vi "SeCrTs-ACC_Read_P3.vi"(7 "Data FIFO Ref":T1, 8 "error in (no error)":errorcluster, 9 "number of samples per channel":i32, 10 "ACC_Task":refnum<k21>) -> (0 "error out":errorcluster, 2 "task out":refnum<k21>)   [LabVIEW 2022 SP3]
uses:
  RT Controls/SeCrTs-Data FIFO.ctl
  <vilib>/Platform/TimedLoop/XDataNode/timing_clust.ctl
  <vilib>/Platform/TimedLoop/XDataNode/nitl_modes.ctl
  <vilib>/Platform/TimedLoop/XDataNode/wakeup.ctl
  <vilib>/DAQmx/read.llb/DAQmx Read (Analog 1D Wfm NChan NSamp).vi
  <vilib>/DAQmx/miscellaneous.llb/DAQmx Fill In Error Info.vi
  <vilib>/platform/TimedLoop/XDataNode/XDataNode.xnode
  <vilib>/Platform/TimedLoop/XDataNode/XDNodeRunTimeDep.lvlib
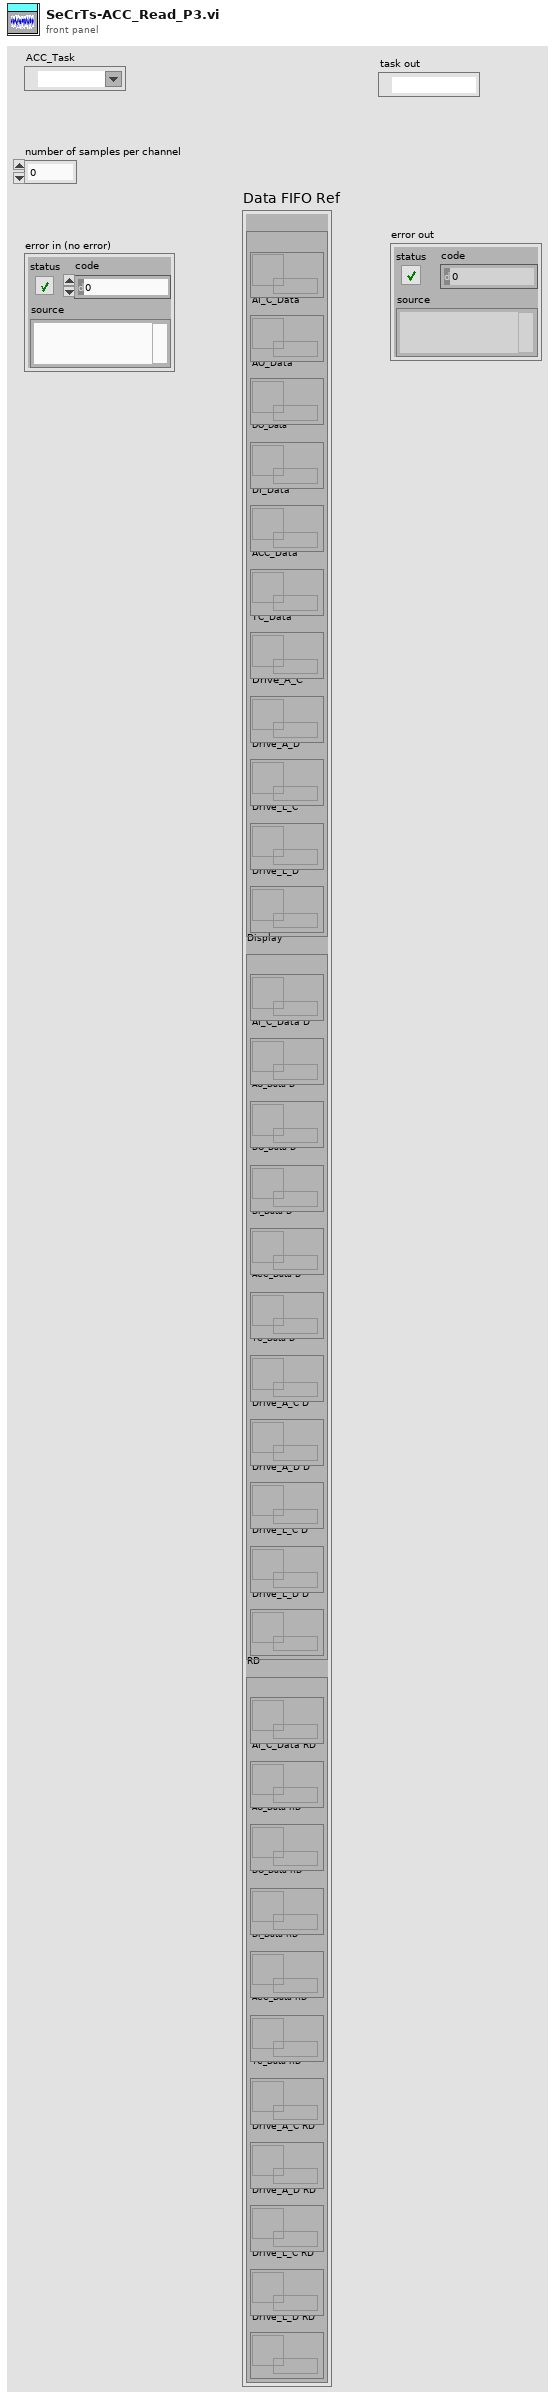
[diagram p1: front panel]
types:
  T1 = typedef "SeCrTs-Data FIFO.ctl" = cluster{"Control":cluster{"AI_V_Data":refnum<queue>, "AI_C_Data":refnum<queue>, "AO_Data":refnum<queue>, "DO_Data":refnum<queue>, "DI_Data":refnum<queue>, "ACC_Data":refnum<queue>, "TC_Data":refnum<queue>, "Drive_A_C":refnum<queue>, "Drive_A_D":refnum<queue>, "Drive_L_C":refnum<queue>, "Drive_L_D":refnum<queue>}, "Display":cluster{"AI_V_Data D":refnum<queue>, "AI_C_Data D":refnum<queue>, "AO_Data D":refnum<queue>, "DO_Data D":refnum<queue>, "DI_Data D":refnum<queue>, "ACC_Data D":refnum<queue>, "TC_Data D":refnum<queue>, "Drive_A_C D":refnum<queue>, "Drive_A_D D":refnum<queue>, "Drive_L_C D":refnum<queue>, "Drive_L_D D":refnum<queue>}, "RD":cluster{"AI_V_Data RD":refnum<queue>, "AI_C_Data RD":refnum<queue>, "AO_Data RD":refnum<queue>, "DO_Data RD":refnum<queue>, "DI_Data RD":refnum<queue>, "ACC_Data RD":refnum<queue>, "TC_Data RD":refnum<queue>, "Drive_A_C RD":refnum<queue>, "Drive_A_D RD":refnum<queue>, "Drive_L_C RD":refnum<queue>, "Drive_L_D RD":refnum<queue>}}
  T2 = typedef "XDNodeRunTimeDep.lvlib/timing_clust.ctl" = cluster{"Expected End [f-1]":u64, "Actual End [f-1]":u64, "Finished Late? [f-1]":bool, "Expected End [i-1]":u64, "Actual End [i-1]":u64, "Finished Late? [i-1]":bool, "Expected Start [i]":u64, "Actual Start [i]":u64, "Expected Start [f]":u64, "Actual Start [f]":u64, "Source Name":string, "Structure Name":string, "Period":i64, "Deadline":i64, "Offset":i64, "Start":i64, "Priority":i32, "Timeout":i32, "Mode":T3, "Wakeup Reason":T4, "Error":errorcluster, "Source Type":string, "Secondary Source Type":string, "Global End Time":u64, "Global Start Time":u64, "Frame Duration":u64, "Iteration Duration":u64, "Assigned CPU":i32, "I/O Scan Engine Mode":u32}
  T3 = typedef "XDNodeRunTimeDep.lvlib/nitl_modes.ctl" = enum32{"No Change", "Process missed periods, maintain original phase", "Discard missed periods, maintain original phase", "Process missed periods, ignore original phase", "Discard missed periods, ignore original phase"}
  T4 = typedef "XDNodeRunTimeDep.lvlib/wakeup.ctl" = enum32{"Normal", "Aborted", "Asynchronous wakeup", "Timing source error", "Timed loop error", "Timeout"}
  T5 = enum16{"Init", "Read 'All'", "Read 'n'", "Read '1'", "Write '1'", "Write 'n'", "Write 'All'"}
  T6 = enum16{"AI C", "AI V", "AO", "DI", "DO", "TC", "ACC", "DR L", "DR A"}
  T7 = cluster{"Start DAQ":bool, "Stop DAQ":bool, "RT Stop":bool, "RT Exit":bool, "Start Seq":bool}
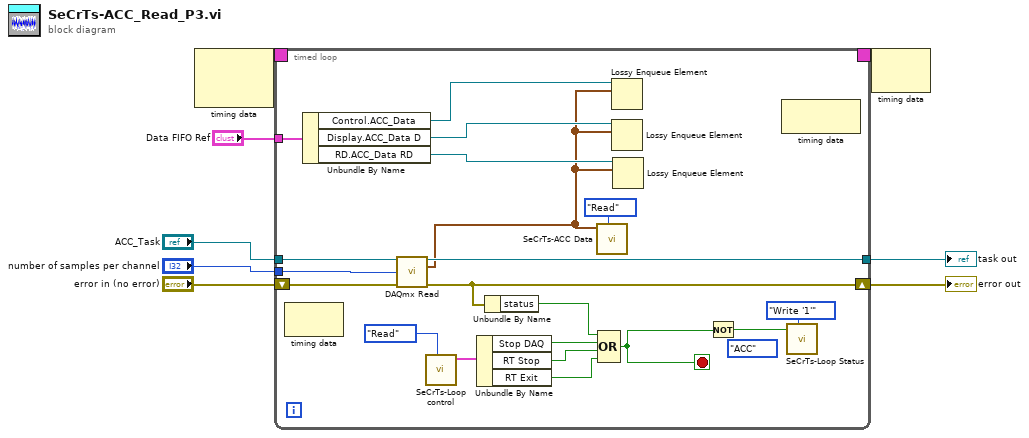
[diagram p0: block diagram]
diagram:
  n1 = node-c288() -> (w8:T2)  [unwired: 2 in]
  n2 = timed-loop {
    shift-right: [w27] -> w2
    shift-left: "error in (no error)" -> [w25]
    tunnel: "ACC_Task" -> [w26]
    tunnel: [w28] -> w5
    tunnel: "number of samples per channel" -> [w24]
    timing: w8 -> [_]
    timing-out: [_] -> w7
    tunnel: "Data FIFO Ref" -> [w16]
    stop <- w10 stop-if-true
    (unwired) T6."ACC" ("Loop")
    n3 = node-c288() -> ()  [unwired: 1 in, 1 out]
    n4 = Unbundle By Name(w16) -> ("Control.ACC_Data"=w15:refnum<queue>, "Display.ACC_Data D"=w14:refnum<queue>, "RD.ACC_Data RD"=w13:refnum<queue>)
    n5 = call-poly <vilib>:"DAQmx Read.vi"("task/channels in"=w26, "number of samples per channel"=w24, "error in"=w25) -> ("task out"=w28:refnum<k21>, "data"=w12:waveform(dbl)[], "error out"=w27:errorcluster)  [unwired: 10 in]
    n6 = call "SeCrTs-Loop control.vi"("Action"=enum16{"Init", "Write", "Read"}."Read") -> ("Loop Control out"=w21:T7)  [unwired: 9 in, 1 out]
    n7 = Unbundle By Name(w21) -> ("Stop DAQ"=w20:bool, "RT Stop"=w19:bool, "RT Exit"=w18:bool)
    n8 = Unbundle By Name(w27) -> ("status"=w23:bool)
    n9 = call "SeCrTs-ACC Data.vi"("Enum"=enum16{"Write", "Read"}."Read", "In_ACC data"=w12) -> ()  [unwired: 9 in, 1 out]
    n10 = Compound Arithmetic op=OR(w23, w20, w19, w18) -> (w10:bool)
    n11 = Lossy Enqueue Element(queue=w15, element=w12) -> ()  [unwired: 1 in, 4 out]
    n12 = Lossy Enqueue Element(queue=w14, element=w12) -> ()  [unwired: 1 in, 4 out]
    n13 = Lossy Enqueue Element(queue=w13, element=w12) -> ()  [unwired: 1 in, 4 out]
    n14 = Not(x=w10) -> (.not. x?=w11:bool)
    n15 = node-c288() -> ()  [unwired: 1 in, 1 out]
    n16 = call "SeCrTs-Loop Status.vi"("Option"=T5."Write '1'", "Status"=w11) -> ()  [unwired: 7 in, 3 out]
  }
  "task out" <- w5
  "error out" <- w2
  n17 = node-c288(w7) -> ()  [unwired: 1 out]
